vi "Write Real Allele.vi"(8 "error in (no error)":errorcluster, 10 "Real Allele":dbl, 11 "Real Gene in":refnum<class "Real Gene.lvclass">) -> (0 "error out":errorcluster, 3 "Real Gene out":refnum<class "Real Gene.lvclass">)   [LabVIEW 2016, in "Real Gene.lvclass"]
uses:
  Real Gene.lvclass
  Real Gene.lvclass/Real Gene.ctl
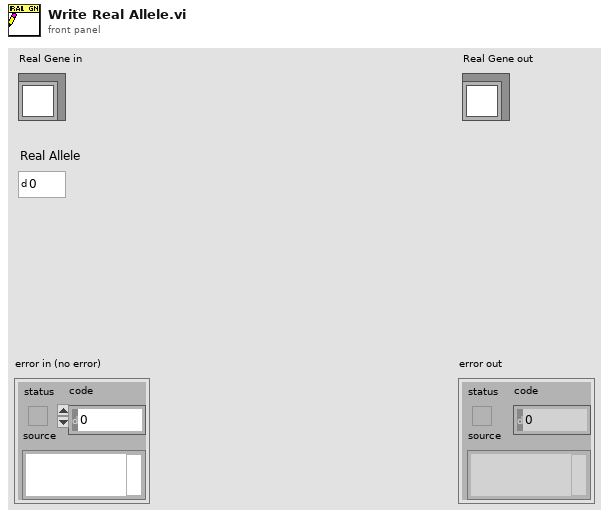
[diagram p1: front panel]
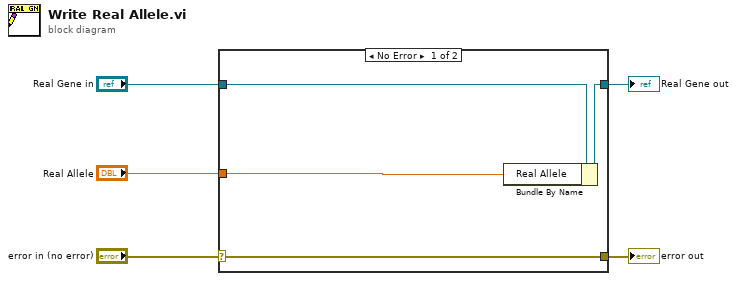
[diagram p0: block diagram]
diagram:
  n1 = case shown="No Error" "error in (no error)" {
    selector: "error in (no error)" -> [w9 w10]
    tunnel: [w9 w10] -> w4
    tunnel: [w7 w11] -> w2
    tunnel: "Real Gene in" -> [w8 w11]
    tunnel: "Real Allele" -> [w6 _]
    frame No Error {
      n2 = Bundle By Name(cluster=w8, "Real Allele"=w6) -> (w7:refnum<class "Real Gene.lvclass">)
    }
    frame Error {
    }
  }
  "error out" <- w4
  "Real Gene out" <- w2
